vi "Initialize System.vi"(7 "Max no of Traces":i32=1000) -> (0 "error out":errorcluster, 2 "Acquired Traces Queue":refnum<queue>, 3 "Next State Queue":refnum<queue>)   [LabVIEW 2019]
uses:
  Controls/DAQ States.ctl
  Controls/Acquisition Result.ctl
  Controls/Global Variable Control.ctl
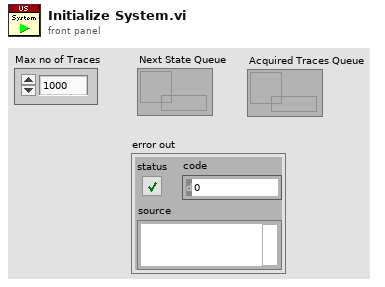
[diagram p1: front panel]
types:
  T1 = typedef "DAQ States.ctl" = enum16{"Initialize", "Idle", "Set Horizontal", "Set Vertical", "Set Trigger", "Set Display", "Acquire", "Analyze", "Set Switch", "Shutdown", "Quit"}
  T2 = typedef "Acquisition Result.ctl" = cluster{"Traces":waveform(sgl)[], "Relative t0 [s]":dbl, "Sample Rate [1/s]":dbl, "No. of points":i32, "Absolute t0 [s]":dbl, "dT [s]":dbl, "Update rate [1/s]":dbl, "Auto Triggered":bool, "Stop":bool}
  T3 = typedef "Global Variable Control.ctl" = enum16{"Clear", "Set", "Get"}
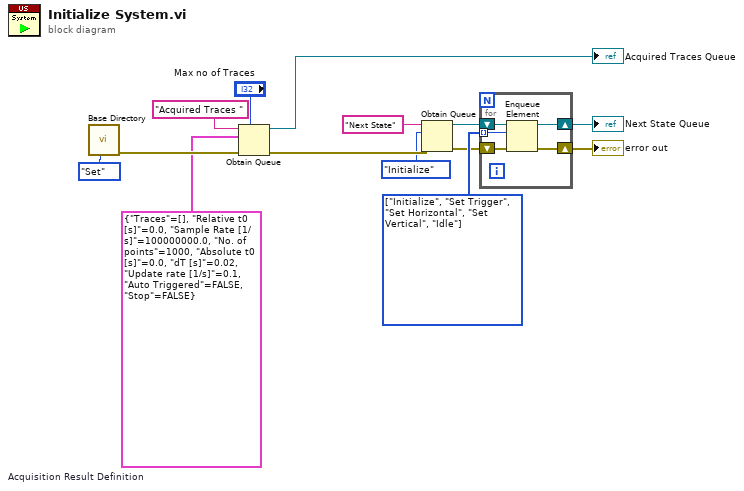
[diagram p0: block diagram]
diagram:
  w5 = T2 {"Traces"=[], "Relative t0 [s]"=0.0, "Sample Rate [1/s]"=100000000.0, "No. of points"=1000, "Absolute t0 [s]"=0.0, "dT [s]"=0.02, "Update rate [1/s]"=0.1, "Auto Triggered"=FALSE, "Stop"=FALSE}  # Acquisition Result Definition
  w11 = T1[] [enum."Initialize", enum."Set Trigger", enum."Set Horizontal", enum."Set Vertical", enum."Idle"] items=["Initialize", "Idle", "Set Horizontal", "Set Vertical", "Set Trigger", "Set Display", "Acquire", "Analyze", "Set Switch", "Shutdown", "Quit"]
  n1 = call "Base Directory.vi"("Operation"=Global_Variable_Control."Set") -> ("Error Out"=w12:errorcluster)  [unwired: 9 in, 1 out]
  n2 = Obtain Queue(max queue size (-1, unlimited)="Max no of Traces", name (unnamed)="Acquired Traces ", element data type=w5, error in (no error)=w12) -> (queue out=→"Acquired Traces Queue":refnum<queue>, error out=w13:errorcluster)  [unwired: 1 in, 1 out]
  n3 = Obtain Queue(name (unnamed)="Next State", element data type=DAQ_States."Initialize", error in (no error)=w13) -> (queue out=w8:refnum<queue>, error out=w9:errorcluster)  [unwired: 2 in, 1 out]
  n4 = for {
    shift-right: [w17] -> w14
    shift-left: w9 -> [w19]
    shift-right: [w18] -> w10
    shift-left: w8 -> [w16]
    tunnel: w11 -> [w15] mode=indexing
    n5 = Enqueue Element(queue=w16, element=w15, error in (no error)=w19) -> (queue out=w18:refnum<queue>, error out=w17:errorcluster)  [unwired: 1 in, 1 out]
  }
  "error out" <- w14
  "Next State Queue" <- w10
